vi "Abort Movement.vi"(8 "error in (no error)":errorcluster) -> (0 "error out":errorcluster)   [LabVIEW 2011]
panel:
  in  "VISA resource name":refnum<visa-resource-name>
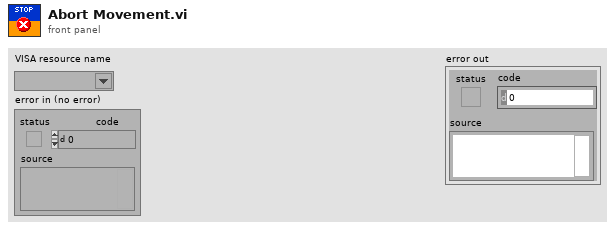
[diagram p1: front panel]
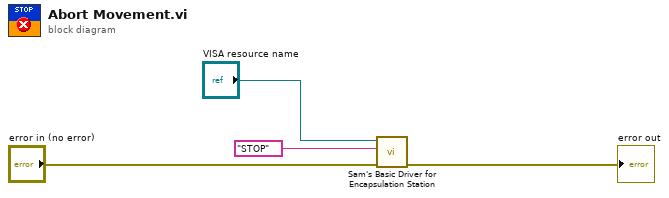
[diagram p0: block diagram]
diagram:
  n1 = call "Sam's Basic Driver for Encapsulation Station.vi"("error in (no error)"="error in (no error)", "Combo Box"="STOP", "VISA resource name"="VISA resource name") -> ("error out"=→"error out":errorcluster)  [unwired: 6 in, 2 out]
